vi "DEMO.vi"() -> ()   [LabVIEW 2012]
uses:
  System.Windows.Forms
  Employee Info/Employee Info.ctl
  LowLevel/DataGridView.lvlib
  Employee Info/Employee Info.lvlib
panel:
  in  "Array":T1[](array[typedef])
  in  "停止":bool
  in  "DataGridView":refnum<k24>(container)
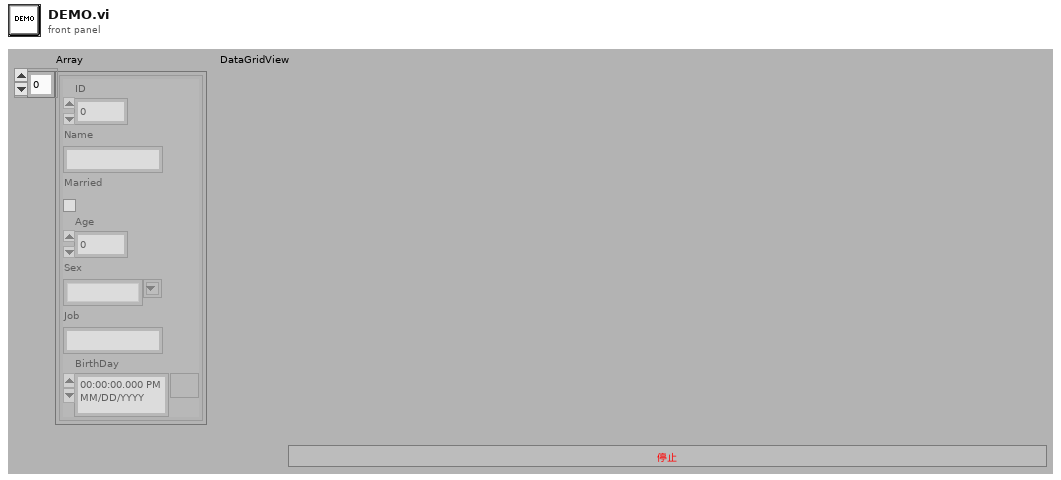
[diagram p1: front panel]
types:
  T1 = typedef "Employee Info.lvlib/Employee Info.ctl" = cluster{"ID":u16, "Name":string, "Married":bool, "Age":u8, "Sex":string, "Job":string, "BirthDay":timestamp}
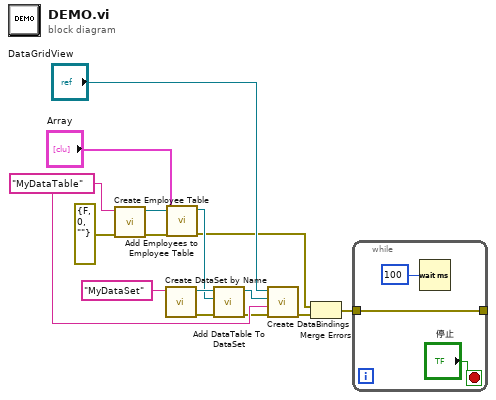
[diagram p0: block diagram]
diagram:
  w11 = "MyDataTable" ("tableName")
  n1 = call "Create Employee Table.vi"("错误输入（无错误）"=errorcluster {"status"=FALSE, "code"=0, "source"=""}, "TableName"=w11) -> ("错误输出"=w5:errorcluster, "DataTable Out"=w4:refnum<k24>)  [unwired: 8 in]
  n2 = call "Create DataSet by Name.vi"("dataSetName"="MyDataSet") -> ("错误输出"=w10:errorcluster, "DataSet Out"=w13:refnum<k24>)  [unwired: 9 in]
  n3 = call "Add Employees to Employee Table.vi"("错误输入（无错误）"=w5, "Array"="Array", "DataTable"=w4) -> ("错误输出（无错误）"=w1:errorcluster, "DataTable Out"=w2:refnum<k24>)  [unwired: 7 in]
  n4 = call "Add DataTable To DataSet.vi"("错误输入（无错误）"=w10, "DataTable"=w2, "DataSet In"=w13) -> ("错误输出"=w9:errorcluster, "DataSet Out"=w12:refnum<k24>)  [unwired: 7 in]
  n5 = call "Create DataBindings.vi"("error in (no error)"=w9, "DataMember"=w11, "dataSource"=w12, "DataGridView"="DataGridView") -> ("error out"=w7:errorcluster)  [unwired: 6 in, 1 out]
  n6 = Merge Errors(w1, w7) -> (w6:errorcluster)
  n7 = while {
    tunnel: w6 -> [w16]
    tunnel: [w16] -> _
    stop <- "停止" stop-if-true
    n8 = Wait (ms)(milliseconds to wait=u32 100 ("等待时间（毫秒）")) -> ()  [unwired: 1 out]
  }
